vi "Install Routine.vi"   [LabVIEW 2013]
uses:
  <vilib>/Utility/sysdir.llb/System Directory Type.ctl
  <vilib>/zip/NI_Unzip.lvlib
panel:
  # "Extracting and placing utility dependencies.\n\n\nPlease wait..."
types:
  T1 = typedef "System Directory Type.ctl" = i32
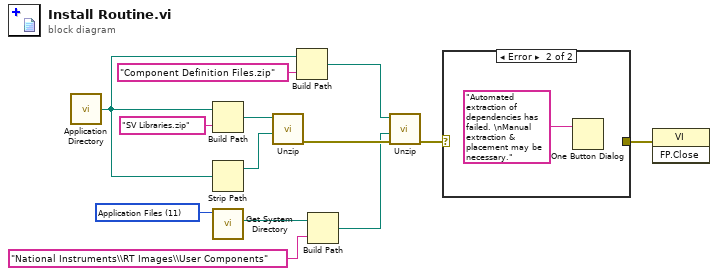
[diagram p0: block diagram]
diagram:
  w13 = T1 11 items=["User Home"=0, "User Desktop"=1, "User Documents"=2, "User Application Data"=3, "User Preferences"=4, "User Temporary"=5, "Public Documents"=6, "Public Application Data"=7, "Public Preferences"=8, "Public Cache"=13, "System Core Libraries"=9, "System Installed Libraries"=10, "Application Files"=11, "Boot Volume Root"=12] ("system directory type")
  n1 = call <vilib>:"Application Directory.vi"() -> ("Application Directory"=w2:path)
  n2 = Build Path(base path=w2, name or relative path="SV Libraries.zip") -> (appended path=w11:path)
  n3 = Strip Path(path=w2) -> (stripped path=w10:path)  [unwired: 1 out]
  n4 = call <vilib>:"Get System Directory.vi"("system directory type"=w13) -> ("system directory"=w6:path)  [unwired: 10 in]
  n5 = call <vilib>:"Unzip.vi"("Target directory (same as Zip file if empty)"=w10, "Zip file"=w11) -> ("error out"=w8:errorcluster)  [unwired: 7 in, 2 out]
  n6 = Build Path(base path=w2, name or relative path="Component Definition Files.zip") -> (appended path=w7:path)
  n7 = Build Path(base path=w6, name or relative path="National Instruments\\RT Images\\User Components") -> (appended path=w4:path)
  n8 = call <vilib>:"Unzip.vi"("error in (no error)"=w8, "Target directory (same as Zip file if empty)"=w4, "Zip file"=w7) -> ("error out"=w3:errorcluster)  [unwired: 6 in, 2 out]
  n9 = case shown="Error" w3 {
    selector: w3 -> [w14 _]
    tunnel: [w14 _] -> w1
    frame No Error {
    }
    frame Error {
      n10 = One Button Dialog(message="Automated extraction of dependencies has failed. \nManual extraction & placement may be necessary.") -> ()  [unwired: 1 in, 1 out]
    }
  }
  n11 = invoke class="VI" method="FP.Close"(error in=w1) -> ()  [unwired: 2 in, 3 out]
